vi "open_matrix.vi"(2 "Numeric":i32) -> (6 "Output Matrix":T1)   [LabVIEW 2019]
uses:
  <vilib>/silver_ctls/ArrayMatrixCluster/Real Matrix NI_Silver.ctl
panel:
  in  "OK Button":bool
  in  "Input Matrix":dbl[][](array[numeric])=[[0.0, 0.0, 0.0]]
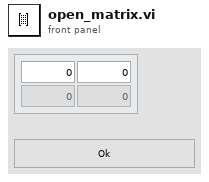
[diagram p1: front panel]
types:
  T1 = typedef "Real Matrix NI_Silver.ctl" = dbl[][]
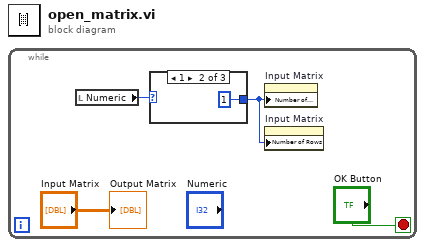
[diagram p0: block diagram]
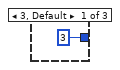
[diagram p2: hidden frame]
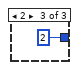
[diagram p3: hidden frame]
diagram:
  n1 = while {
    stop <- "OK Button" stop-if-true
    n2 = local read "Numeric"() -> (w2:i32)
    n3 = case shown="1" w2 {
      tunnel: [u32 3 ("Number of Columns") u32 1 ("Number of Columns") u32 2 ("Number of Columns")] -> w1
      frame 3, Default {
      }
      frame 1 {
      }
      frame 2 {
      }
    }
    n4 = property on="Input Matrix" class="Arr (strict)"("Number of Columns"=w1) -> ()  [unwired: 2 in, 2 out]
    n5 = property on="Input Matrix" class="Arr (strict)"("Number of Rows"=w1) -> ()  [unwired: 2 in, 2 out]
    "Output Matrix" <- "Input Matrix"
  }
